vi "ECG Feauture Extractor(SubVI).vi"(9 "Array":T1[](array[typedef]), 10 "data":dynamicdata(waveform), 11 "Denoised Signal":waveform(dbl)) -> (2 "Statistics":T2, 3 "Array of Features":T1[](array[typedef]))   [LabVIEW 2024]
uses:
  <vilib>/addons/Biomedical/Biosignal Measurements/ECG/subVIs/ECG features.ctl
  <vilib>/addons/Biomedical/Biosignal Measurements/ECG/subVIs/ecg feature params in.ctl
  <vilib>/addons/Biomedical/Biosignal Measurements/ECG/subVIs/ecg feature param selector.ctl
  <vilib>/addons/Biomedical/Biosignal Measurements/ECG/subVIs/ecg qrs params in.ctl
  <vilib>/addons/Biomedical/Biosignal Measurements/ECG/ECG Feature Extractor (Waveform All).vi
  <vilib>/addons/Biomedical/NI_BMTK_Measurements.lvlib
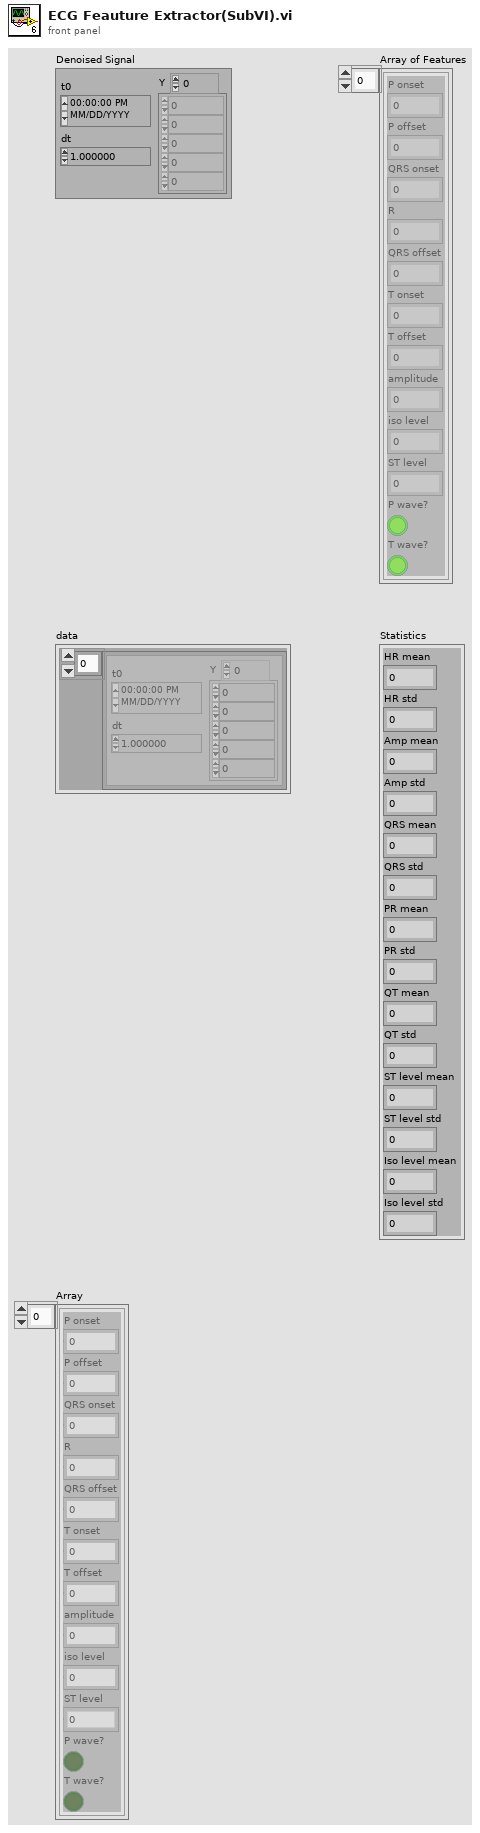
[diagram p1: front panel]
types:
  T1 = typedef "NI_BMTK_Measurements.lvlib/ECG features.ctl" = cluster{"P onset":dbl, "P offset":dbl, "QRS onset":dbl, "R":dbl, "QRS offset":dbl, "T onset":dbl, "T offset":dbl, "amplitude":dbl, "iso level":dbl, "ST level":dbl, "P wave?":bool, "T wave?":bool}
  T2 = cluster{"HR mean":dbl, "HR std":dbl, "Amp mean":dbl, "Amp std":dbl, "QRS mean":dbl, "QRS std":dbl, "PR mean":dbl, "PR std":dbl, "QT mean":dbl, "QT std":dbl, "ST level mean":dbl, "ST level std":dbl, "Iso level mean":dbl, "Iso level std":dbl}
  T3 = typedef "NI_BMTK_Measurements.lvlib/ecg qrs params in.ctl" = cluster{"threshold factor":dbl, "freq bands":cluster{"low":dbl, "high":dbl}, "QRS onset offset":cluster{"QRS onset":T4, "QRS offset":T4}}
  T4 = typedef "NI_BMTK_Measurements.lvlib/ecg feature param selector.ctl" = i32
  T5 = typedef "NI_BMTK_Measurements.lvlib/ecg feature params in.ctl" = cluster{"isoelectric limit":dbl, "PR interval":T4, "QT interval":T4}
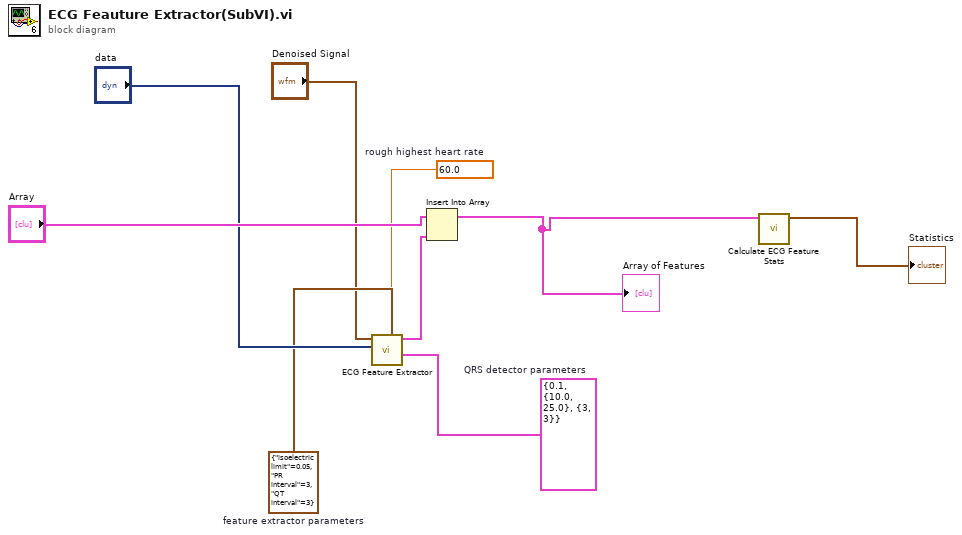
[diagram p0: block diagram]
diagram:
  w1 = 60.0 items=["500 bpm"=500.0, "300 bpm"=300.0, "200 bpm"=200.0, "150 bpm"=150.0, "100 bpm"=100.0, "60 bpm"=60.0, "20 bpm"=20.0, "10 bpm"=10.0]  # rough highest heart rate
  w4 = T3 {"threshold factor"=0.1, "freq bands"={"low"=10.0, "high"=25.0}, "QRS onset offset"={"QRS onset"=3, "QRS offset"=3}}  # QRS detector parameters
  w3 = T5 {"isoelectric limit"=0.05, "PR interval"=3, "QT interval"=3}  # feature extractor parameters
  n1 = call-poly <vilib>:"ECG Feature Extractor.vi"("feature extractor parameters"=w3, "rough highest heart rate"=w1, "QRS detector parameters"=w4, "raw ECG"="data", "ECG"="Denoised Signal") -> ("ECG features"=w6:T1[])  [unwired: 5 in, 1 out]
  n2 = Insert Into Array "Insert Into Array"(array="Array", new element=w6) -> (w8:T1[])  [unwired: 1 in]
  "Array of Features" <- w8
  n3 = call "Calculate ECG Feature Stats.vi"("ECG Features"=w8) -> ("Statistics"=→"Statistics":T2)  [unwired: 10 in]
